vi "MUX_CommandsGlobal.vi"() -> ()   [LabVIEW 2013, in "Switching.lvclass"]
uses:
  Switching.lvclass
panel:
  in  "Pickering MUX GPIB Setup":T1={"Mux1 address"="4", "Mux2 address"="5", "Instrument name"="Pickering MUX", "Instrument type"=2, "Command \"MUX Reset\""="areset %s", "Command \"Select MUX Channel\""="CH %d,%d,%d"} {"Instrument type" items=["Supply", "LCR", "Switching"]}
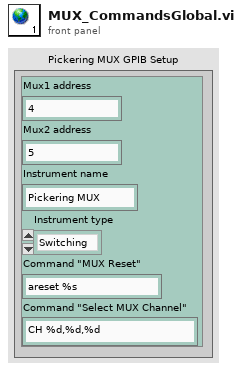
[diagram p1: front panel]
types:
  T1 = cluster{"Mux1 address":string, "Mux2 address":string, "Instrument name":string, "Instrument type":u16, "Command \"MUX Reset\"":string, "Command \"Select MUX Channel\"":string}
diagram:
